vi "Load JSON Configuration for Interactive Testing.vi"(8 "error in (no error)":errorcluster, 10 "Configuration JSON":string, 11 "CIFTemplateNode in":refnum<class "CIFCorePlugin.lvclass">) -> (0 "error out":errorcluster, 3 "CIFTemplateNode out":refnum<class "CIFCorePlugin.lvclass">)   [LabVIEW 2021, in "CIFCorePlugin.lvclass"]
uses:
  CIFCorePlugin.lvclass
  CIFCorePlugin.lvclass/CIFCorePlugin.ctl
  CIFUtilities/CIFOutOfBand/CIFOutOfBand.lvclass/CIFOutOfBand.ctl
  CIFUtilities/CIFOutOfBand/Accessors/Read Local OOB Data.vi
  CIFUtilities/CIFOutOfBand/Write OOB DVR.vi
  CIFUtilities/CIFOutOfBand/Accessors/Write Local OOB Data.vi
  CIFUtilities/CIFOutOfBand/Utilities/Command to Bitwise Command.vi
  CIFUtilities/CIFOutOfBand/Read OOB DVR.vi
  OOB/OOB_Rx/Private/Command Settings.vi
  OOB/OOB_Rx/CIFCoreOOB_Rx.lvclass
  D:/dev/CIF-LVCore/src/CIFUtilities/CIFOutOfBand/CIFOutOfBand.lvclass
  <vilib>/addons/_JKI.lib/Serialization/JSON/Library/Unflatten From JSON String.vi
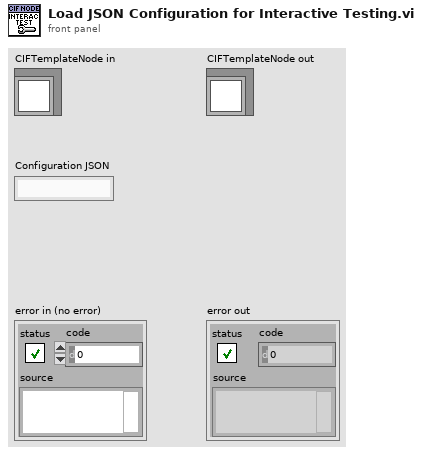
[diagram p1: front panel]
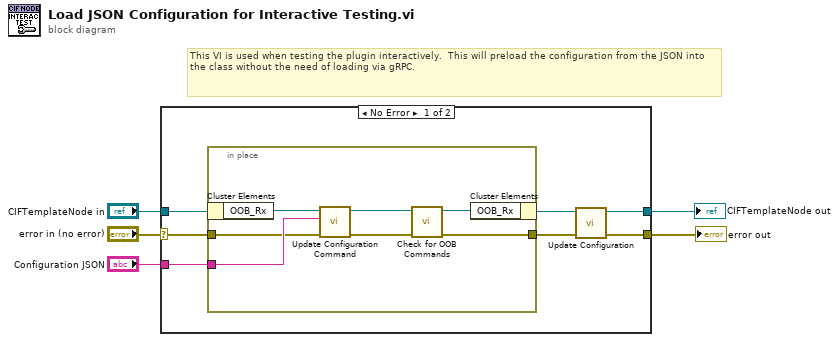
[diagram p0: block diagram]
diagram:
  # "This VI is used when testing the plugin interactively.  This will preload the configuration from the JSON into the class without the need of loading via gRPC."
  n1 = case shown="No Error" "error in (no error)" {
    selector: "error in (no error)" -> [w11 w20]
    tunnel: [w7 w20] -> w4
    tunnel: [w6 w21] -> w2
    tunnel: "CIFTemplateNode in" -> [w12 w21]
    tunnel: "Configuration JSON" -> [w10 _]
    frame No Error {
      n2 = in-place {
        in-place-border: w11 -> [w17]
        in-place-border: w10 -> [w19]
        in-place-border: [w13] -> w8
        n3 = in-place-cluster #1(w12) -> ("OOB_Rx"=w18:refnum<class "CIFCoreOOB_Rx.lvclass">)
        n4 = call "Update Configuration Command.vi"("error in"=w17, "Config JSON"=w19, "CoreOOB_Rx in"=w18) -> ("error out"=w15:errorcluster, "CoreOOB_Rx out"=w16:refnum<class "CIFCoreOOB_Rx.lvclass">)  [unwired: 7 in]
        n5 = call "Check for OOB Commands.vi"("error in (no error)"=w15, "CoreOOB_Rx in"=w16) -> ("error out"=w13:errorcluster, "CoreOOB_Rx out"=w14:refnum<class "CIFCoreOOB_Rx.lvclass">)  [unwired: 6 in, 2 out]
        n6 = in-place-cluster #1("OOB_Rx"=w14) -> (w9:refnum<class "CIFCorePlugin.lvclass">)
      }
      n7 = call-dynamic "Update Configuration.vi"("error in (no error)"=w8, "CIFTemplateNode in"=w9) -> ("error out"=w7:errorcluster, "CIFTemplateNode out"=w6:refnum<class "CIFCorePlugin.lvclass">)  [unwired: 8 in]
    }
    frame Error {
    }
  }
  "error out" <- w4
  "CIFTemplateNode out" <- w2
